vi "Format Data into Table.vi"(8 "error in (no error)":errorcluster, 9 "Passed?":bool[](array[boolean]), 10 "Signals":dynamicdata(waveform), 11 "Tbl Refnum":refnum<vi>) -> (0 "error out":errorcluster, 2 "Table":string[][](array[string]), 3 "Tbl Refnum Out":refnum<vi>)   [LabVIEW 2012]
uses:
  <vilib>/Utility/miscctls.llb/LVRowAndColumnTypeDef.ctl
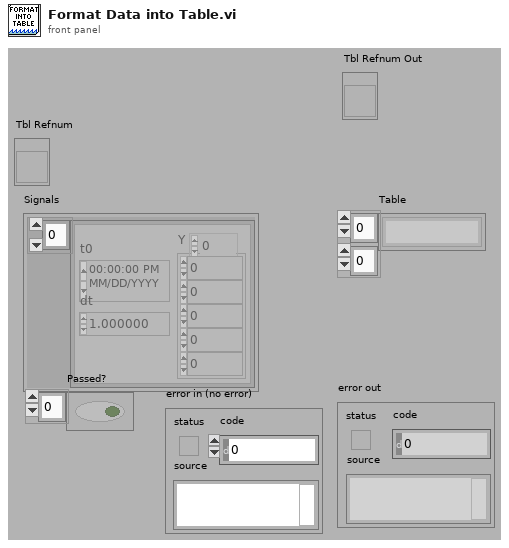
[diagram p1: front panel]
types:
  T1 = typedef "LVRowAndColumnTypeDef.ctl" = cluster{"Row":i32, "Column":i32}
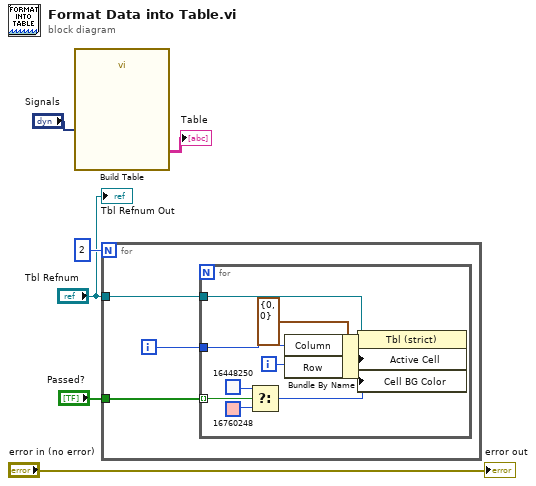
[diagram p0: block diagram]
diagram:
  n1 = call "Build Table"("Signals"="Signals") -> ("Table"=→"Table":string[][])  [unwired: 9 in, 1 out]
  n2 = for {
    N: 2 -> [_]
    tunnel: "Passed?" -> [w9]
    tunnel: "Tbl Refnum" -> [w7]
    i -> [w8]
    n3 = for {
      tunnel: w9 -> [w16] mode=indexing
      tunnel: w8 -> [w13]
      tunnel: w7 -> [w10]
      i -> [w14]
      n4 = Select(t=u32 16448250, s=w16, f=u32 16760248) -> (s? t:f=w15:u32)
      n5 = Bundle By Name(cluster=T1 {"Row"=0, "Column"=0} ("Active Cell:Active Cell"), "Column"=w13, "Row"=w14) -> (w17:T1)
      n6 = property on="Property Node" class="Tbl (strict)"(reference=w10, "Active Cell"=w17, "Cell BG Color"=w15) -> ()  [unwired: 1 in, 2 out]
    }
  }
  "Tbl Refnum Out" <- "Tbl Refnum"
  "error out" <- "error in (no error)"
